vi "switchToStreamMode.vi"(8 "error in (no error)":errorcluster, 9 "Stream Mode Algorithm":T1, 10 "model":refnum<class "Model.lvclass">, 11 "DataOnDemandState in":refnum<class "DataOnDemandState.lvclass">) -> (0 "error out":errorcluster, 2 "model 2":refnum<class "Model.lvclass">, 3 "DataOnDemandState out":refnum<class "DataOnDemandState.lvclass">)   [LabVIEW 2013, in "DataOnDemandState.lvclass"]
uses:
  DataOnDemandState.lvclass
  Model/Model/Model.lvclass
  Configuration/Stream Mode Algorithm.ctl
  Typedefs/StateSelector.ctl
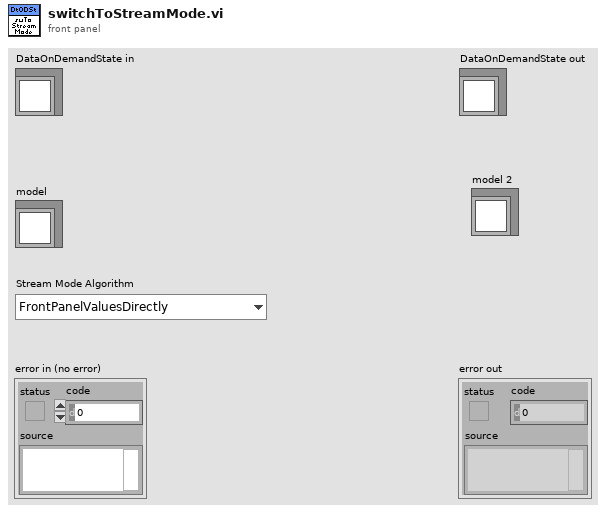
[diagram p1: front panel]
types:
  T1 = typedef "Stream Mode Algorithm.ctl" = enum16{"FrontPanelValuesDirectly"}
  T2 = typedef "StateSelector.ctl" = enum16{"DataOnDemandState", "DataStreamingState", "FaultState", "OffState", "StandbyState"}
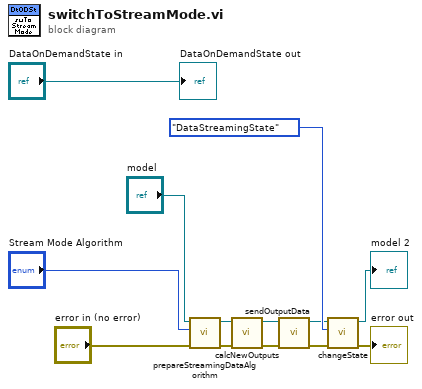
[diagram p0: block diagram]
diagram:
  n1 = call "prepareStreamingDataAlgorithm.vi"("error in (no error)"="error in (no error)", "Stream Mode Algorithm"="Stream Mode Algorithm", "Model in"="model") -> ("error out"=w4:errorcluster, "Model out"=w5:refnum<class "Model.lvclass">)  [unwired: 7 in]
  n2 = call "calcNewOutputs.vi"("error in (no error)"=w4, "Model in"=w5) -> ("error out"=w6:errorcluster, "Model out"=w3:refnum<class "Model.lvclass">)  [unwired: 8 in]
  n3 = call "sendOutputData.vi"("error in (no error)"=w6, "Model in"=w3) -> ("error out"=w1:errorcluster, "Model out"=w2:refnum<class "Model.lvclass">)  [unwired: 8 in]
  n4 = call "changeState.vi"("error in (no error)"=w1, "State:"=StateSelector."DataStreamingState", "Model in"=w2) -> ("error out"=→"error out":errorcluster, "Model out"=→"model 2":refnum<class "Model.lvclass">)  [unwired: 7 in]
  "DataOnDemandState out" <- "DataOnDemandState in"
